vi "destroy c Daq .vi"(11 "handle":u32) -> (2 "function return":bool, 3 "handle out":u32)   [LabVIEW 2020, in "cDaq.lvlib"]
doc: "DAQAPI bool destroy_cDaq_(HDAQ handle);"
uses:
  cDaq.lvlib
  <userlib>/cDaq/cDaq.dll
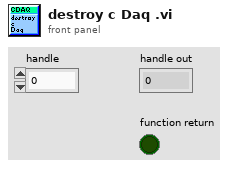
[diagram p1: front panel]
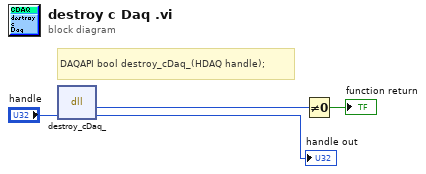
[diagram p0: block diagram]
diagram:
  # "DAQAPI bool destroy_cDaq_(HDAQ handle);"
  n1 = dll-call lib="C:/Program Files (x86)/National Instruments/LabVIEW 2020/user.lib/cDaq/cDaq.*" fn="destroy_cDaq_"("handle"="handle") -> ("type de retour"=w3:u8, "handle"=→"handle out":u32)  [unwired: 3 in, 2 out]
  n2 = Not Equal To 0?(x=w3) -> (x != 0?=→"function return":bool)
